vi "Init.vi"(8 "error in (no error)":errorcluster, 9 "SequenceCountService":refnum<class "SequenceCountService.lvclass">, 10 "ChannelService":refnum<class "ChannelService.lvclass">) -> (0 "error out":errorcluster, 3 "RemoteDataService out":refnum<class "RemoteDataService.lvclass">)   [LabVIEW 2020, in "Vecto.lvlib" / "RemoteDataService.lvclass"]
uses:
  RemoteDataService.lvclass
  Publish Group Data.ctl
  proto/GroupData/Class/Msg.lvclass
  ChannelService/ChannelService.lvclass
  SequenceCountService/SequenceCountService.lvclass
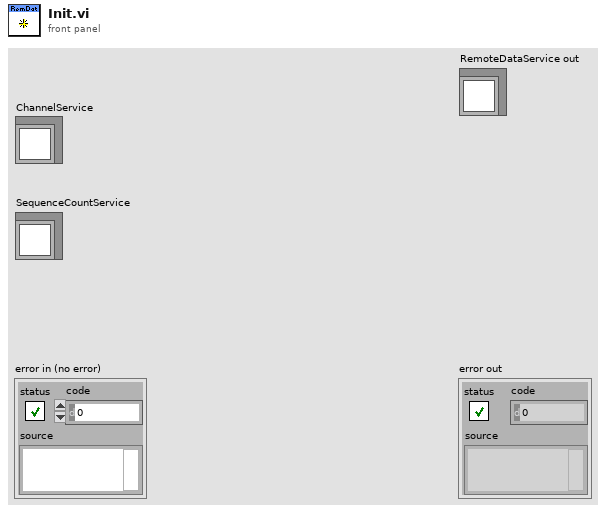
[diagram p1: front panel]
types:
  T1 = typedef "Vecto.lvlib/RemoteDataService.lvclass/Publish Group Data.ctl" = cluster{"GroupData":refnum<class "Msg.lvclass">}
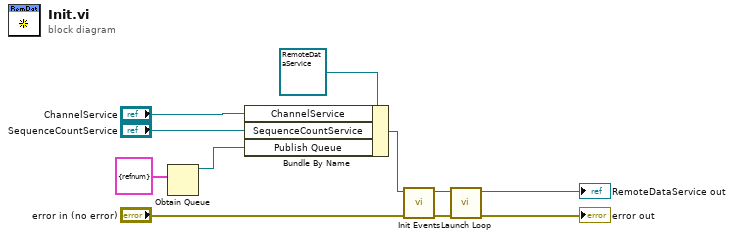
[diagram p0: block diagram]
diagram:
  n1 = Obtain Queue(element data type=T1 {"GroupData"=refnum} ("Publish Group Data")) -> (queue out=w1:refnum<queue>)  [unwired: 4 in, 2 out]
  n2 = Bundle By Name(cluster=refnum<class "RemoteDataService.lvclass"> refnum ("RemoteDataService in"), "ChannelService"="ChannelService", "SequenceCountService"="SequenceCountService", "Publish Queue"=w1) -> (w7:refnum<class "RemoteDataService.lvclass">)
  n3 = call "Init Events.vi"("error in (no error)"="error in (no error)", "RemoteDataService in"=w7) -> ("error out"=w8:errorcluster, "RemoteDataService out"=w4:refnum<class "RemoteDataService.lvclass">)  [unwired: 8 in]
  n4 = call "Launch Loop.vi"("error in (no error)"=w8, "RemoteDataService in"=w4) -> ("error out"=→"error out":errorcluster, "RemoteDataService out"=→"RemoteDataService out":refnum<class "RemoteDataService.lvclass">)  [unwired: 8 in]
